vi "Mutate_SerializableData_Path.vi"(8 "error in (no error)":errorcluster, 10 "LVClass library Path":path, 11 "class reference":refnum<vi>) -> (0 "error out":errorcluster)   [LabVIEW 2019, in "BlueSerializationScripts.lvlib"]
uses:
  BlueSerializationScripts.lvlib
  UserAppLibs/IncrementMutationHistory/IncrementBlueSerVersionAction.ctl
  <vilib>/Utility/error.llb/Error Cluster From Error Code.vi
  <vilib>/ErrorRing/Error Ring.xnode
  BlueUtilityScripts/BlueUtilityScripts.lvlib
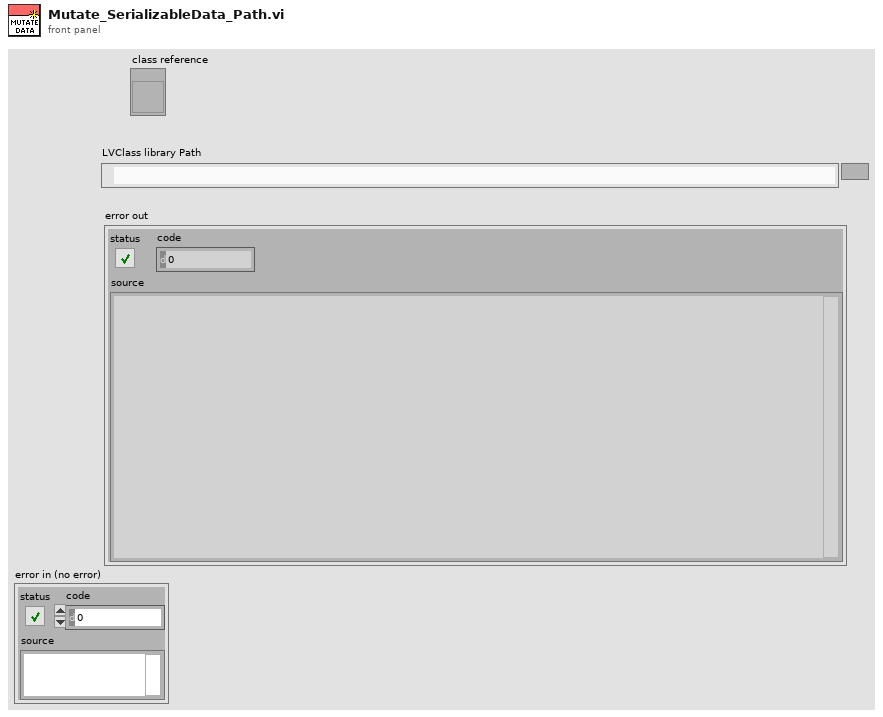
[diagram p1: front panel]
types:
  T1 = typedef "BlueSerializationScripts.lvlib/IncrementBlueSerVersionAction.ctl" = enum16{"Init", "Increment"}
  T2 = typedef "BlueSerializationScripts.lvlib/BlueSerializableTemplatePaths.ctl" = cluster{"GetSerializableData.vi":path, "SerializableData.ctl":path, "SetSerializableData.vi":path, "GetVersionSerializableData.vi":path, "HandleVersionMutation.vi":path, "Mutate_Template.vi":path}
  T3 = typedef "BlueSerializationScripts.lvlib/BlueSerializableMutationPaths.ctl" = cluster{"SerializableData_v2.ctl":path, "Mutate_v1_to_v2.vi":path, "Mutate_v2_to_v3.vi":path}
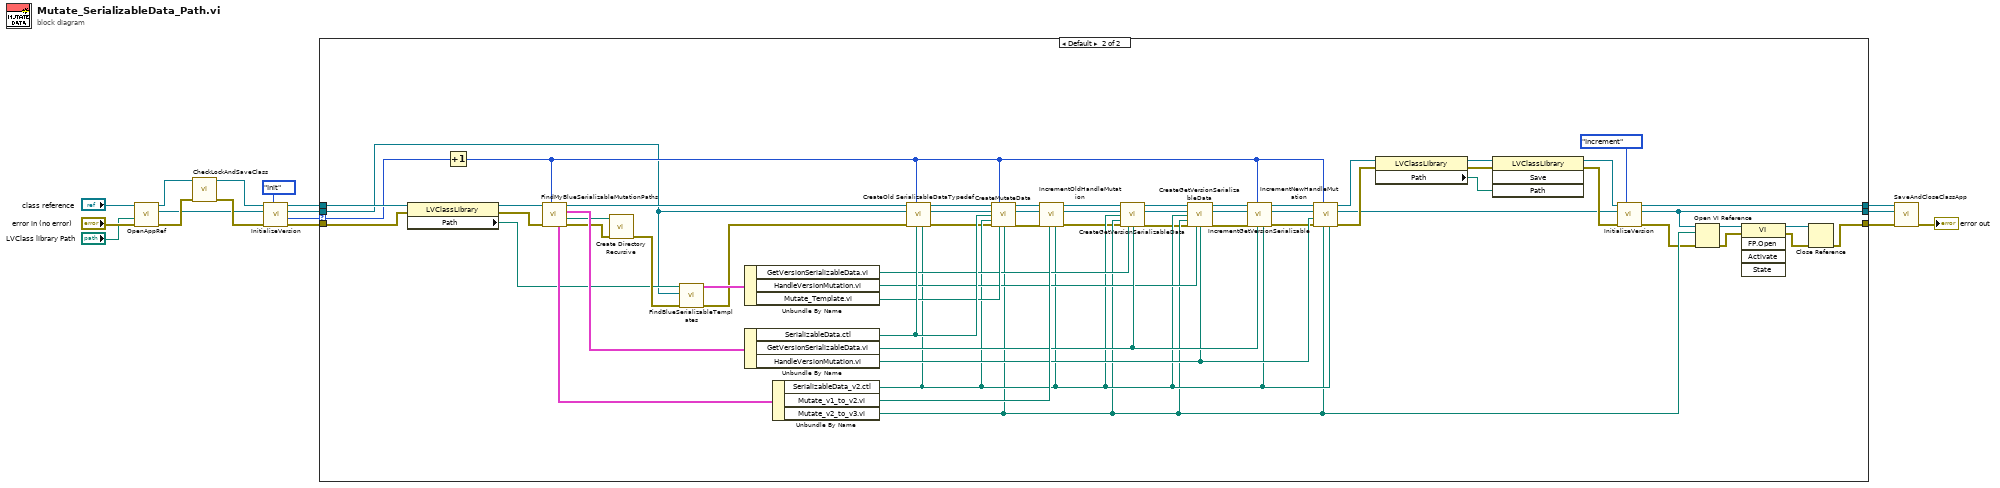
[diagram p0: block diagram]
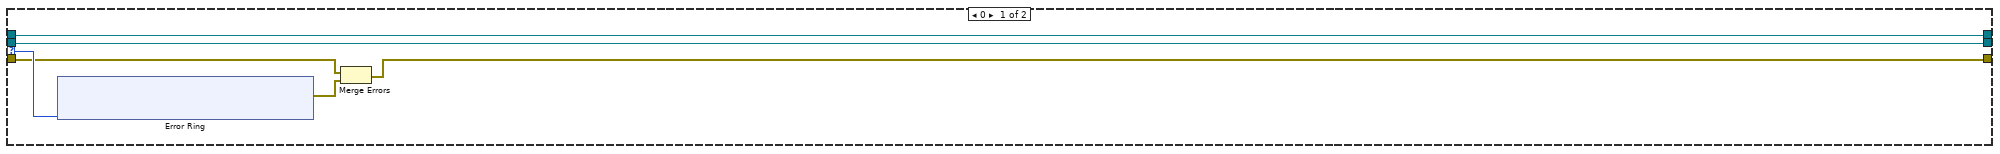
[diagram p2: hidden frame]
diagram:
  n1 = call "OpenAppRef.vi"("error in (no error)"="error in (no error)", "LVClass library Path"="LVClass library Path", "class reference"="class reference") -> ("error out"=w13:errorcluster, "Application reference"=w9:refnum<vi>, "LVClass Reference"=w14:refnum<vi>)  [unwired: 6 in]
  n2 = call "CheckLockAndSaveClass.vi"("error in (no error)"=w13, "LVClass ref"=w14) -> ("error out"=w11:errorcluster, "LVClass ref"=w10:refnum<vi>)  [unwired: 8 in]
  n3 = call "InitializeVersion.vi"("Action"=IncrementBlueSerVersionAction."Init", "error in (no error)"=w11, "Application"=w9, "LVClass ref"=w10) -> ("error out"=w5:errorcluster, "BlueSerializableVersion"=w7:u16, "Application"=w6:refnum<vi>, "LVClass ref"=w8:refnum<vi>)  [unwired: 4 in]
  n4 = case shown="Default" w7 {
    selector: w7 -> [w21 w65]
    tunnel: w8 -> [w23 w66]
    tunnel: w6 -> [w22 w63]
    tunnel: w5 -> [w20 w61]
    tunnel: [w23 w59] -> w4
    tunnel: [w22 w58] -> w3
    tunnel: [w18 w57] -> w2
    frame 0 {
      n5 = xnode "Error Ring"("parameter 0"=w21) -> ("error out"=w19:errorcluster)
      n6 = Merge Errors(w20, w19) -> (w18:errorcluster)
    }
    frame Default {
      n7 = property class="LVClassLibrary"(reference=w66, error in=w61) -> (reference out=w62:refnum<vi>, error out=w60:errorcluster, "Path"=w64:path)
      n8 = Increment(x=w65) -> (x+1=w81:u16)
      n9 = call "FindMyBlueSerializableMutationPaths.vi"("New BlueSerializableVersion"=w81, "error in (no error)"=w60, "LVClass refnum"=w62) -> ("error out"=w86:errorcluster, "BlueSerialization\\Mutations Folder"=w87:path, "BlueSerializable Paths"=w88:T2, "LVClass refnum (dup)"=w75:refnum<vi>, "Mutation Paths"=w85:T3)  [unwired: 4 in]
      n10 = call <vilib>:"Create Directory Recursive.vi"("error in (no error)"=w86, "directory"=w87) -> ("error out"=w89:errorcluster)  [unwired: 3 in, 2 out]
      n11 = call "FindBlueSerializableTemplates.vi"("error in (no error)"=w89, "App Reference (this app)"=w63, "LabVIEW Class Path"=w64) -> ("error out"=w74:errorcluster, "BlueSerializableTemplate Paths"=w90:T2)  [unwired: 7 in]
      n12 = Unbundle By Name(w90) -> ("GetVersionSerializableData.vi"=w80:path, "HandleVersionMutation.vi"=w78:path, "Mutate_Template.vi"=w82:path)
      n13 = Unbundle By Name(w88) -> ("SerializableData.ctl"=w83:path, "GetVersionSerializableData.vi"=w79:path, "HandleVersionMutation.vi"=w77:path)
      n14 = Unbundle By Name(w85) -> ("SerializableData_v2.ctl"=w76:path, "Mutate_v1_to_v2.vi"=w84:path, "Mutate_v2_to_v3.vi"=w67:path)
      n15 = call "CreateOld SerializableDataTypedef.vi"("SerializableData_v2.ctl"=w76, "SerializableData.ctl path"=w83, "New BlueSerializableVersion"=w81, "error in (no error)"=w74, "Application"=w63, "LVClassLibrary Ref"=w75) -> ("error out"=w71:errorcluster, "Application"=w72:refnum<vi>, "LVClassLibrary Ref"=w73:refnum<vi>)  [unwired: 3 in]
      n16 = call "CreateMutateData.vi"("LVClassLibrary Ref"=w73, "New BlueSerializableVersion"=w81, "Application"=w72, "SerializableData.ctl path"=w83, "SerializableData_v2.ctl"=w76, "error in (no error)"=w71, "Mutate_Template.vi path"=w82, "Mutate_SaveTo_Path"=w67) -> ("LVClassLibrary Ref"=w69:refnum<vi>, "Application"=w68:refnum<vi>, "error out"=w70:errorcluster)  [unwired: 5 in]
      n17 = call "IncrementOldHandleMutation.vi"("SerializableData_v2.ctl"=w76, "Mutate_v1_to_v2.vi"=w84, "error in (no error)"=w70, "Application"=w68, "LVClassLibrary Ref"=w69) -> ("error out"=w41:errorcluster, "Application"=w42:refnum<vi>, "LVClassLibrary Ref"=w43:refnum<vi>)  [unwired: 4 in]
      n18 = call "CreateGetVersionSerializableData.vi"("LVClassLibrary Ref"=w43, "Application"=w42, "SerializableData_v2.ctl path"=w76, "Mutate_v2_to_v3.vi path"=w67, "error in (no error)"=w41, "Template VI path"=w80, "SaveTo Path"=w79) -> ("LVClassLibrary Ref"=w46:refnum<vi>, "Application"=w45:refnum<vi>, "error out"=w44:errorcluster)  [unwired: 6 in]
      n19 = call "CreateGetVersionSerializableData.vi"("LVClassLibrary Ref"=w46, "Application"=w45, "SerializableData_v2.ctl path"=w76, "Mutate_v2_to_v3.vi path"=w67, "error in (no error)"=w44, "Template VI path"=w78, "SaveTo Path"=w77) -> ("LVClassLibrary Ref"=w40:refnum<vi>, "Application"=w39:refnum<vi>, "error out"=w38:errorcluster)  [unwired: 6 in]
      n20 = call "IncrementGetVersionSerializable.vi"("SerializableData_v2.ctl"=w76, "GetVersionSerializableData.vi"=w79, "New BlueSerializableVersion"=w81, "error in (no error)"=w38, "Application"=w39, "LVClassLibrary Ref"=w40) -> ("error out"=w54:errorcluster, "Application"=w55:refnum<vi>, "LVClassLibrary Ref"=w56:refnum<vi>)  [unwired: 3 in]
      n21 = call "IncrementNewHandleMutation.vi"("SerializableData_v2.ctl"=w76, "Mutate_v2_to_v3.vi"=w67, "New BlueSerializableVersion"=w81, "error in (no error)"=w54, "HandleVersionMutation.vi"=w77, "Application"=w55, "LVClassLibrary Ref"=w56) -> ("error out"=w49:errorcluster, "Application"=w31:refnum<vi>, "LVClassLibrary Ref"=w50:refnum<vi>)  [unwired: 2 in]
      n22 = property class="LVClassLibrary"(reference=w50, error in=w49) -> (reference out=w52:refnum<vi>, error out=w51:errorcluster, "Path"=w47:path)
      n23 = invoke class="LVClassLibrary" method="Save"(reference=w52, error in=w51, "Path"=w47) -> (reference out=w32:refnum<vi>, error out=w48:errorcluster)  [unwired: 1 in, 2 out]
      n24 = call "InitializeVersion.vi"("Action"=IncrementBlueSerVersionAction."Increment", "error in (no error)"=w48, "Application"=w31, "LVClass ref"=w32) -> ("error out"=w37:errorcluster, "Application"=w58:refnum<vi>, "LVClass ref"=w59:refnum<vi>)  [unwired: 4 in, 1 out]
      n25 = Open VI Reference(application reference (local)=w58, vi path=w67, error in (no error)=w37) -> (vi reference=w36:refnum<vi>, error out=w34:errorcluster)  [unwired: 3 in]
      n26 = invoke class="VI" method="FP.Open"(reference=w36, error in=w34) -> (reference out=w35:refnum<vi>, error out=w33:errorcluster)  [unwired: 3 in, 3 out]
      n27 = Close Reference(reference=w35, error in (no error)=w33) -> (error out=w57:errorcluster)
    }
  }
  n28 = call "SaveAndCloseClassApp.vi"("error in (no error)"=w2, "Application"=w3, "LVClassLibrary Ref"=w4) -> ("error out"=→"error out":errorcluster)  [unwired: 8 in]
